vi "SwissSPAD Live_Sensor Size.vi"(6 "Set/Get(F)":bool, 8 "Error In":errorcluster, 9 "Y size":i32=256, 11 "X size":i32=512) -> (0 "Error Out":errorcluster, 1 "Y size":i32=256, 3 "X size":i32=512)   [LabVIEW 2021]
uses:
  <vilib>/Utility/error.llb/Error Cluster From Error Code.vi
  <vilib>/ErrorRing/Error Ring.xnode
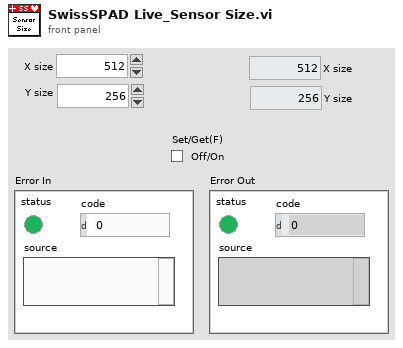
[diagram p1: front panel]
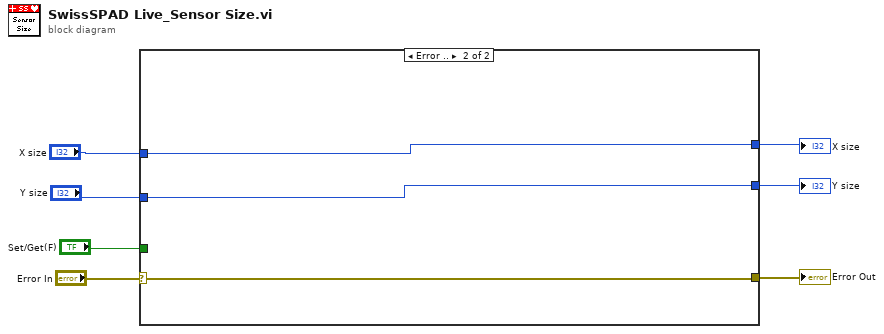
[diagram p0: block diagram]
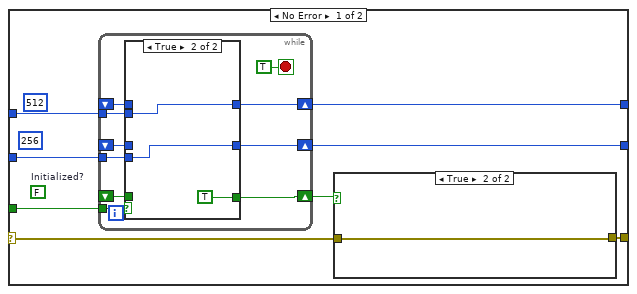
[diagram p2: hidden frame]
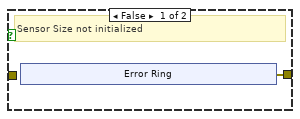
[diagram p3: hidden frame]
diagram:
  n1 = case shown="Error .." "Error In" {
    selector: "Error In" -> [w9 w38]
    tunnel: "Set/Get(F)" -> [w15 _]
    tunnel: "X size" -> [w14 w40]
    tunnel: [w13 w40] -> w5
    tunnel: "Y size" -> [w12 w39]
    tunnel: [w11 w39] -> w3
    tunnel: [w8 w38] -> w1
    frame No Error {
      (unwired) 256 ("Y size")
      (unwired) 512 ("X size")
      (unwired) FALSE  # Initialized?
      n2 = while {
        shift-right: [w30] -> w13
        shift-left: _ -> [w26]
        shift-right: [w28] -> w11
        shift-left: _ -> [w25]
        tunnel: w15 -> [w31]
        tunnel: w14 -> [w29]
        tunnel: w12 -> [w27]
        shift-right: [w23] -> w10
        shift-left: _ -> [w22]
        stop <- TRUE stop-if-true
        n3 = case shown="True" w31 {
          tunnel: [w34 w37] -> w30
          tunnel: w29 -> [_ w37]
          tunnel: [w33 w36] -> w28
          tunnel: w27 -> [_ w36]
          tunnel: w26 -> [w34 _]
          tunnel: w25 -> [w33 _]
          tunnel: [w32 TRUE] -> w23
          tunnel: w22 -> [w32 _]
          frame False {
          }
          frame True {
          }
        }
      }
      n4 = case shown="True" w10 {
        tunnel: w9 -> [_ w21]
        tunnel: [w16 w21] -> w8
        frame False {
          # "Sensor Size not initialized"
          n5 = xnode "Error Ring"() -> ("error out"=w16:errorcluster)
        }
        frame True {
        }
      }
    }
    frame Error {
    }
  }
  "X size" <- w5
  "Y size" <- w3
  "Error Out" <- w1
